vi "Autonomous Independent.vi"   [LabVIEW 2017]
doc: "This VI is called when autonomous begins, and will automatically be terminated when autonomous ends. You can carry out timed or sensor driven robot movement independently without needing to return to the caller."
uses:
  <vilib>/Rock Robotics/WPI/Solenoid/WPI_SolenoidValue.ctl
  <vilib>/Rock Robotics/WPI/SafetyOutput/WPI_SafetyOutputConfigMenu.ctl
  <vilib>/Rock Robotics/WPI/Utilities/WPI_GetSetVariantRefNum.vi
  <vilib>/Rock Robotics/WPI/Solenoid/WPI_SolenoidSetEnum.vi
  <vilib>/Rock Robotics/WPI/RobotDrive/WPI_RobotDriveArcadeDrive_Standard(NoSaturation).vi
  <vilib>/Rock Robotics/Network Tables/NT Read String.vi
  <vilib>/Rock Robotics/Network Tables/NT Write Numeric Array.vi
panel:
  # "Be sure to right-click and choose Data Operations>>Make Current Value default if you want to save the array values with the VI"
types:
  T1 = typedef "WPI_JoystickDevRef.ctl" = cluster{"Device":T2}
  T2 = typedef "WPI_JoystickDeviceEnum.ctl" = enum16{"USB 0", "USB 1", "USB 2", "USB 3", "USB 4", "USB 5"}
  T3 = typedef "WPI_SolenoidDevRef.ctl" = cluster{"DevStatus":errorcluster, "Pneumatics Control Module":u8, "Forward Solenoid Channel":T4, "Reverse Solenoid Channel":T4}
  T4 = typedef "WPI_SolenoidChannel.ctl" = enum8{"Solenoid 0", "Solenoid 1", "Solenoid 2", "Solenoid 3", "Solenoid 4", "Solenoid 5", "Solenoid 6", "Solenoid 7", "Invalid"}
  T5 = typedef "WPI_MotorControlDeviceRef.ctl" = cluster{"DeviceStatus":errorcluster, "Type":T6, "PWM":cluster{"PWM Channel":T7, "DeadBand":T8}, "CAN":cluster{"Device Number":u8, "SetOutput VI Ref":variant, "GetOutput VI Ref":variant, "Enable VI Ref":variant, "Disable VI Ref":variant, "Data":variant}, "Invert":bool, "DIO PWM":cluster{"PWM \"Enable\" Channel":T7, "DIOChannel":T9, "PWM Rate":dbl}}
  T6 = typedef "WPI_MotorControlType.ctl" = enum16{"PWM", "CAN", "DIO PWM"}
  T7 = typedef "FPGA_DIOPWMChannel.ctl" = enum8{"PWM 0", "PWM 1", "PWM 2", "PWM 3", "PWM 4", "PWM 5", "PWM 6", "PWM 7", "PWM 8", "PWM 9", "PWM MXP 0", "PWM MXP 1", "PWM MXP 2", "PWM MXP 3", "PWM MXP 4", "PWM MXP 5", "PWM MXP 6", "PWM MXP 7", "PWM MXP 8", "PWM MXP 9", "Invalid"}
  T8 = typedef "WPI_PWMDeadband.ctl" = cluster{"Name":string, "maxPositivePwm":i32, "minPositivePwm":i32, "centerPwm":i32, "maxNegativePwm":i32, "minNegativePwm":i32, "angularRange":u16}
  T9 = typedef "FPGA_DIOChannel.ctl" = enum8{"DIO 0", "DIO 1", "DIO 2", "DIO 3", "DIO 4", "DIO 5", "DIO 6", "DIO 7", "DIO 8", "DIO 9", "DIO MXP 0", "DIO MXP 1", "DIO MXP 2", "DIO MXP 3", "DIO MXP 4", "DIO MXP 5", "DIO MXP 6", "DIO MXP 7", "DIO MXP 8", "DIO MXP 9", "DIO MXP 10", "DIO MXP 11", "DIO MXP 12", "DIO MXP 13", "DIO MXP 14", "DIO MXP 15", "SPI Port CS1", "SPI Port CS2", "SPI Port CS3", "SPI Port MISO", "SPI Port MOSI", "Invalid"}
  T10 = typedef "WPI_RobotDriveDevRef.ctl" = cluster{"DevStatus":errorcluster, "Motors[]":T5[], "Square Inputs":bool, "Max Output":dbl}
  T11 = typedef "WPI_SolenoidValue.ctl" = enum16{"Off", "On", "Forward", "Reverse"}
  T12 = typedef "WPI_SafetyOutputConfigMenu.ctl" = enum16{"Enable", "Disable"}
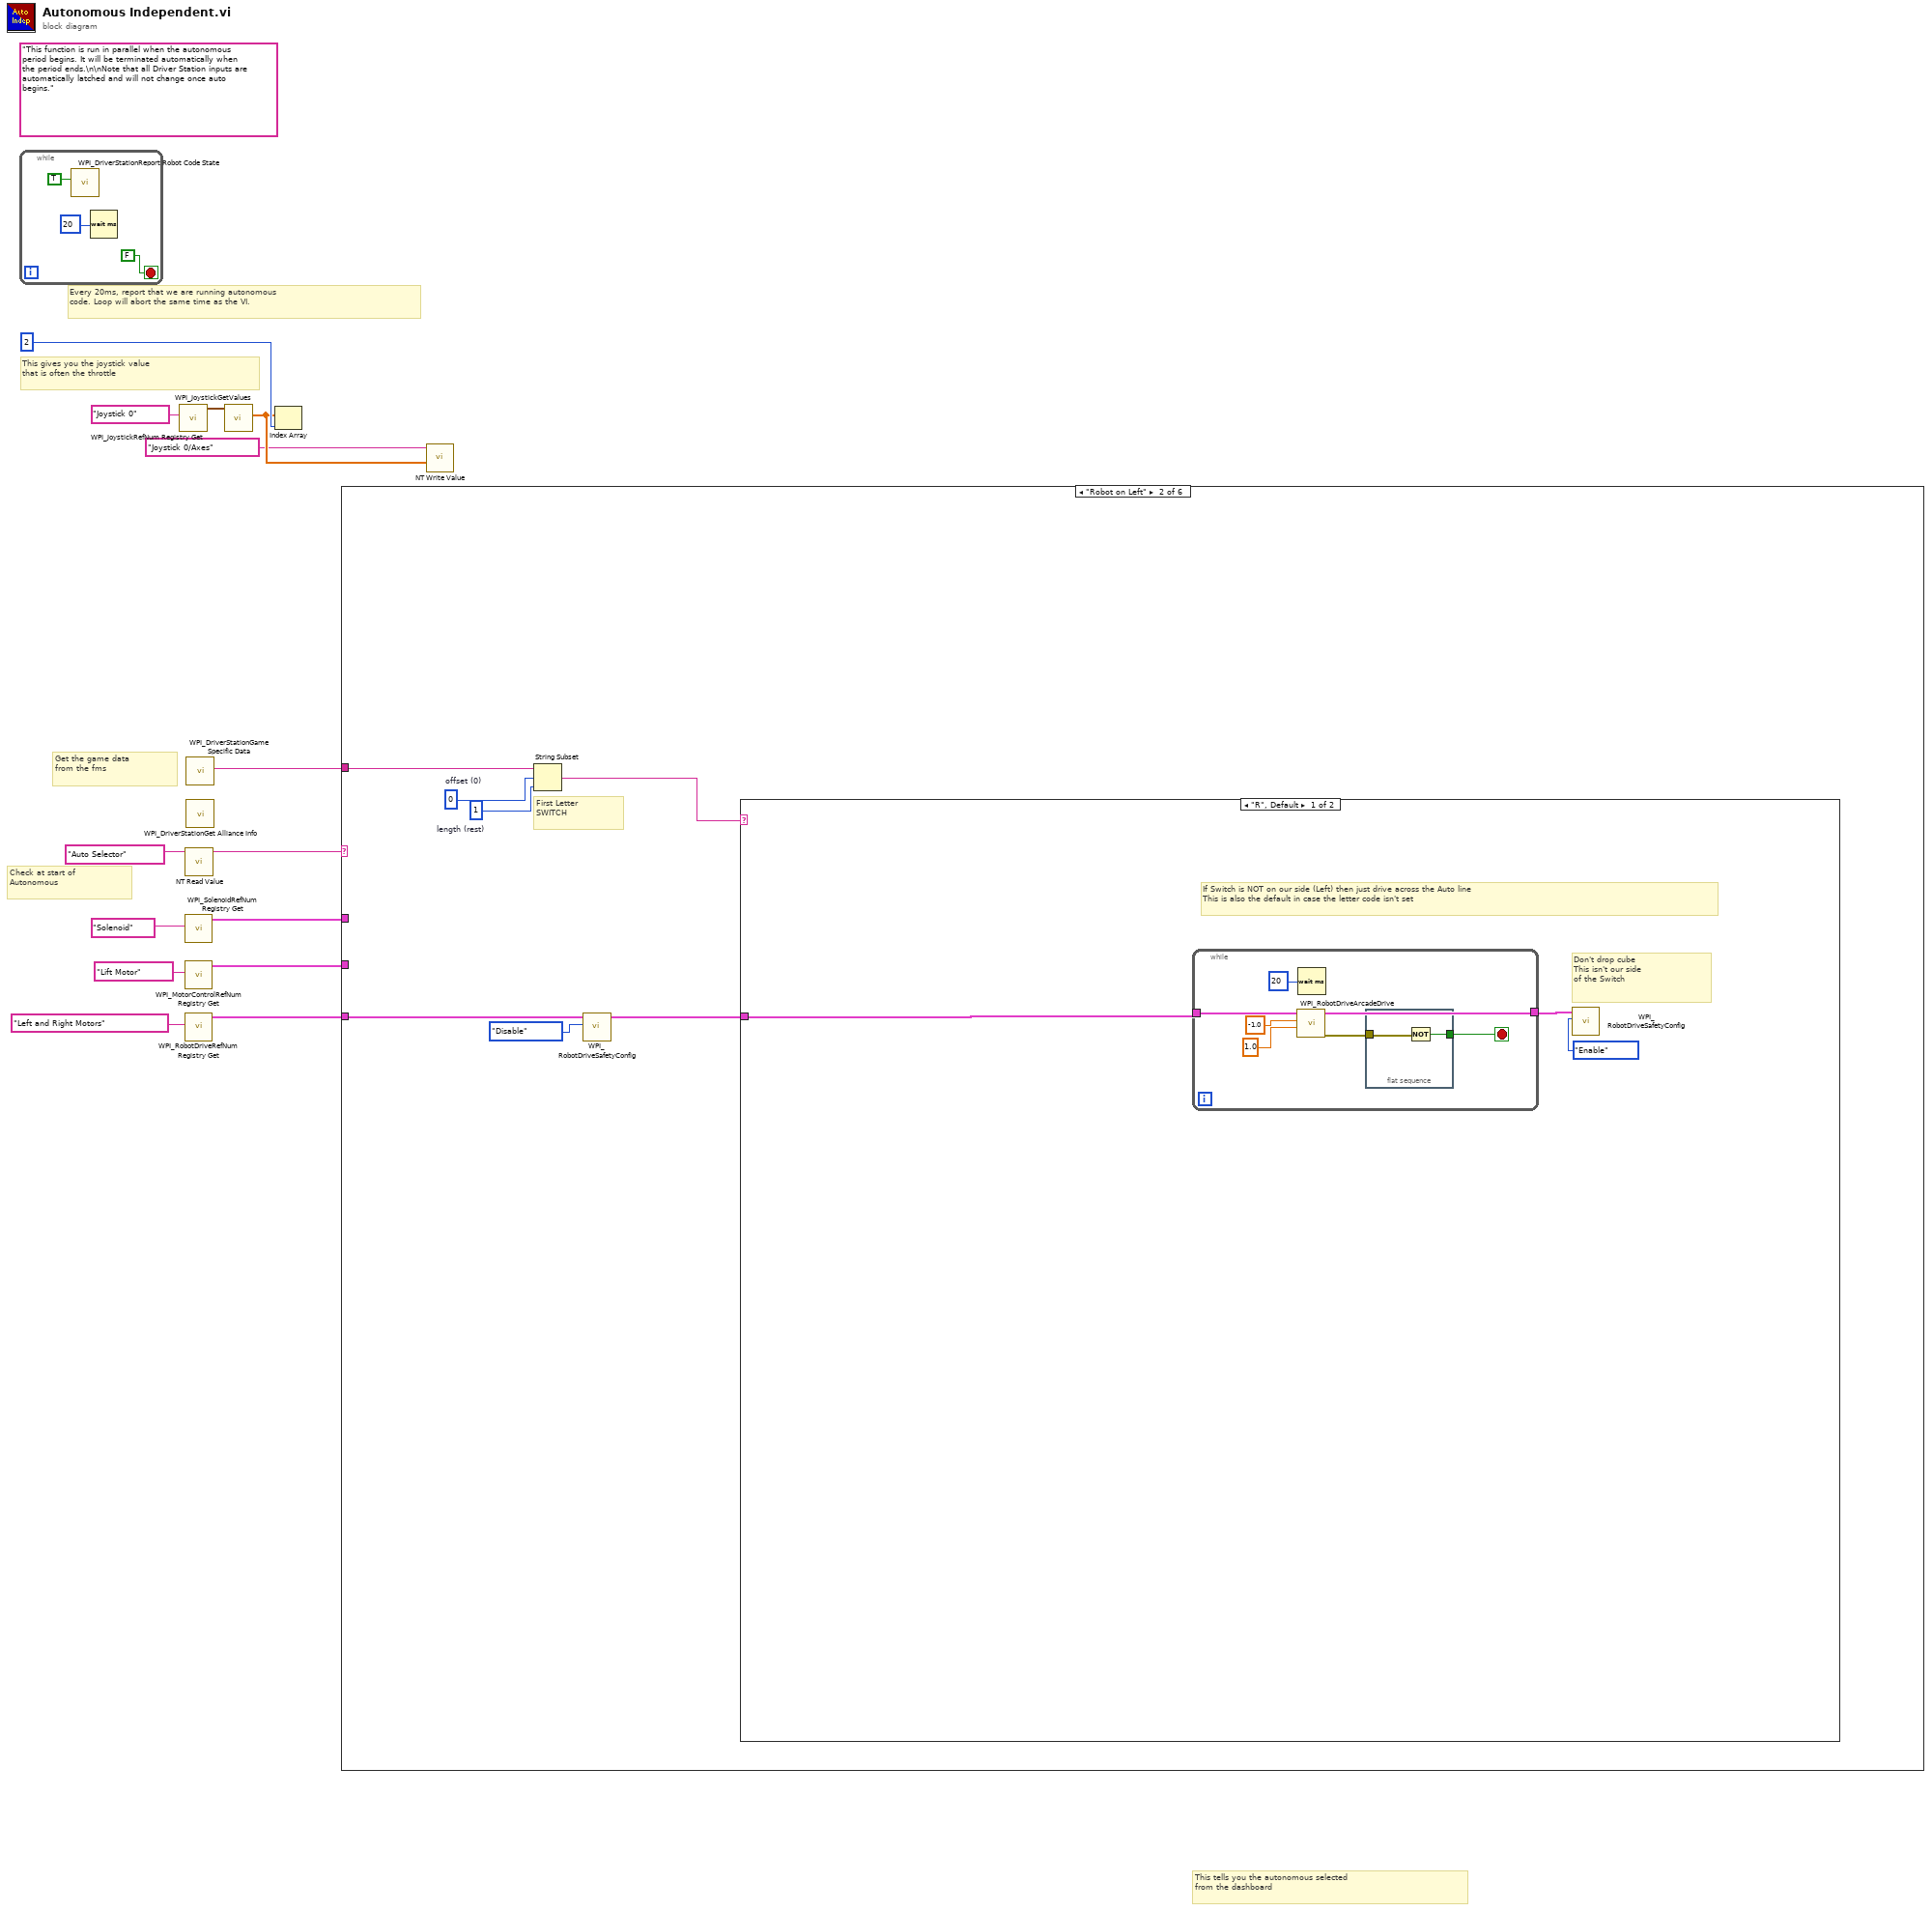
[diagram p0: block diagram]
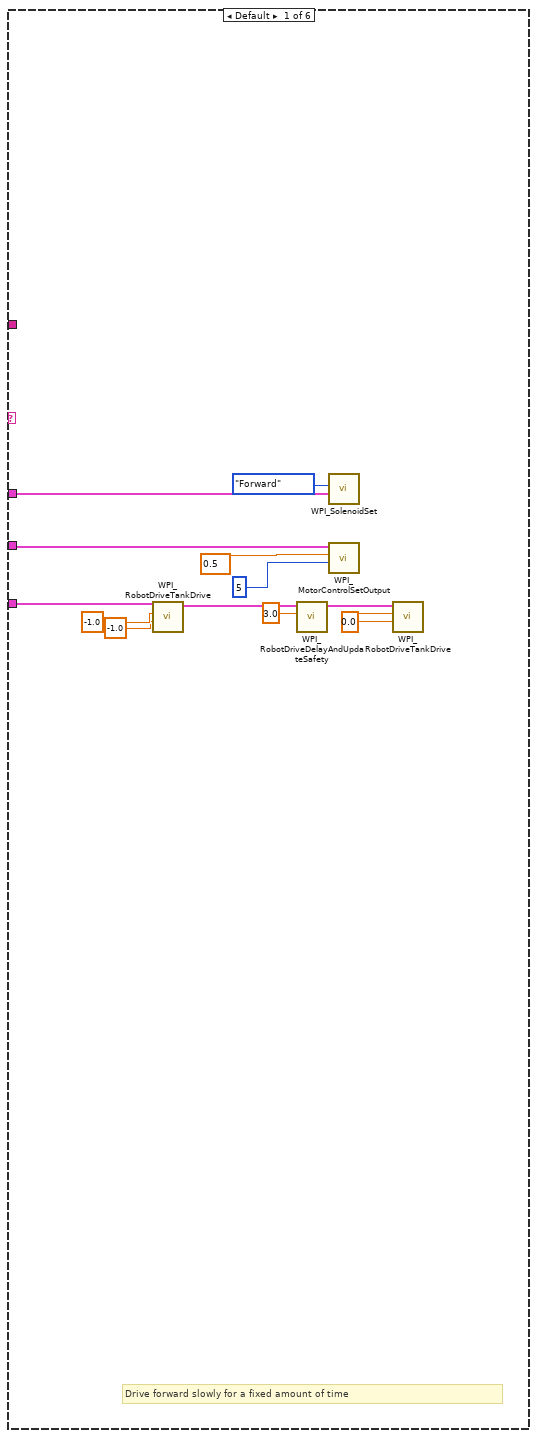
[diagram p2: hidden frame]
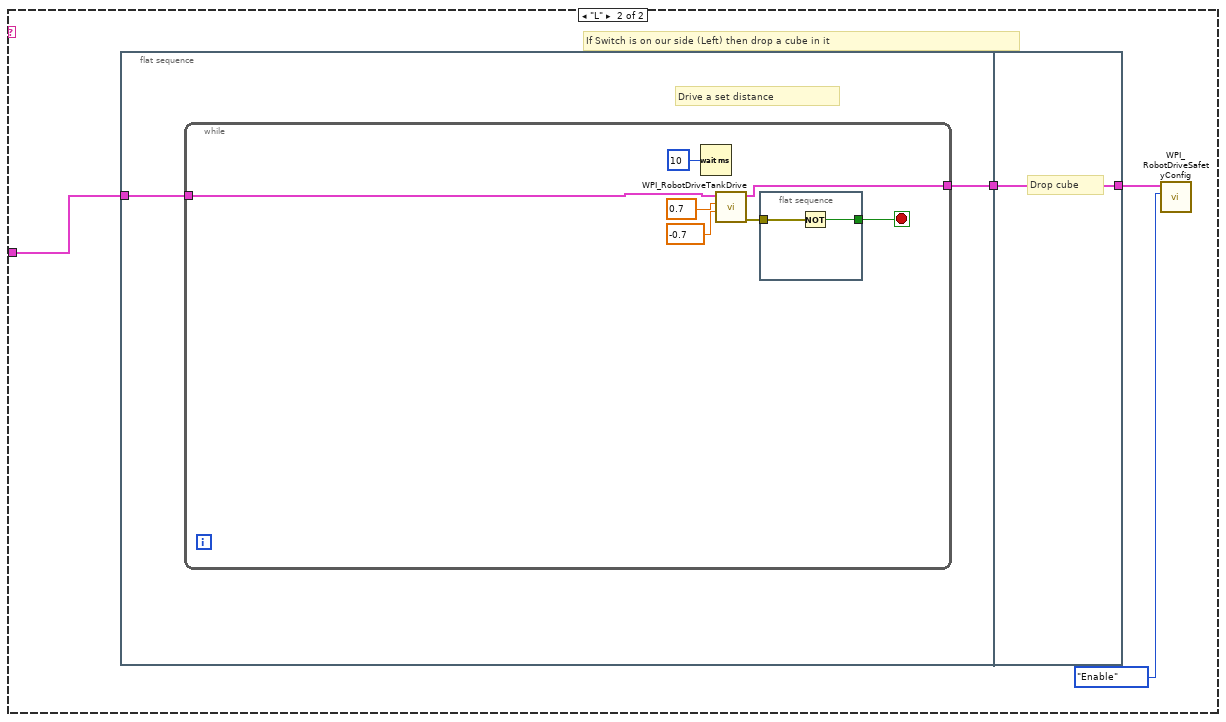
[diagram p3: hidden frame]
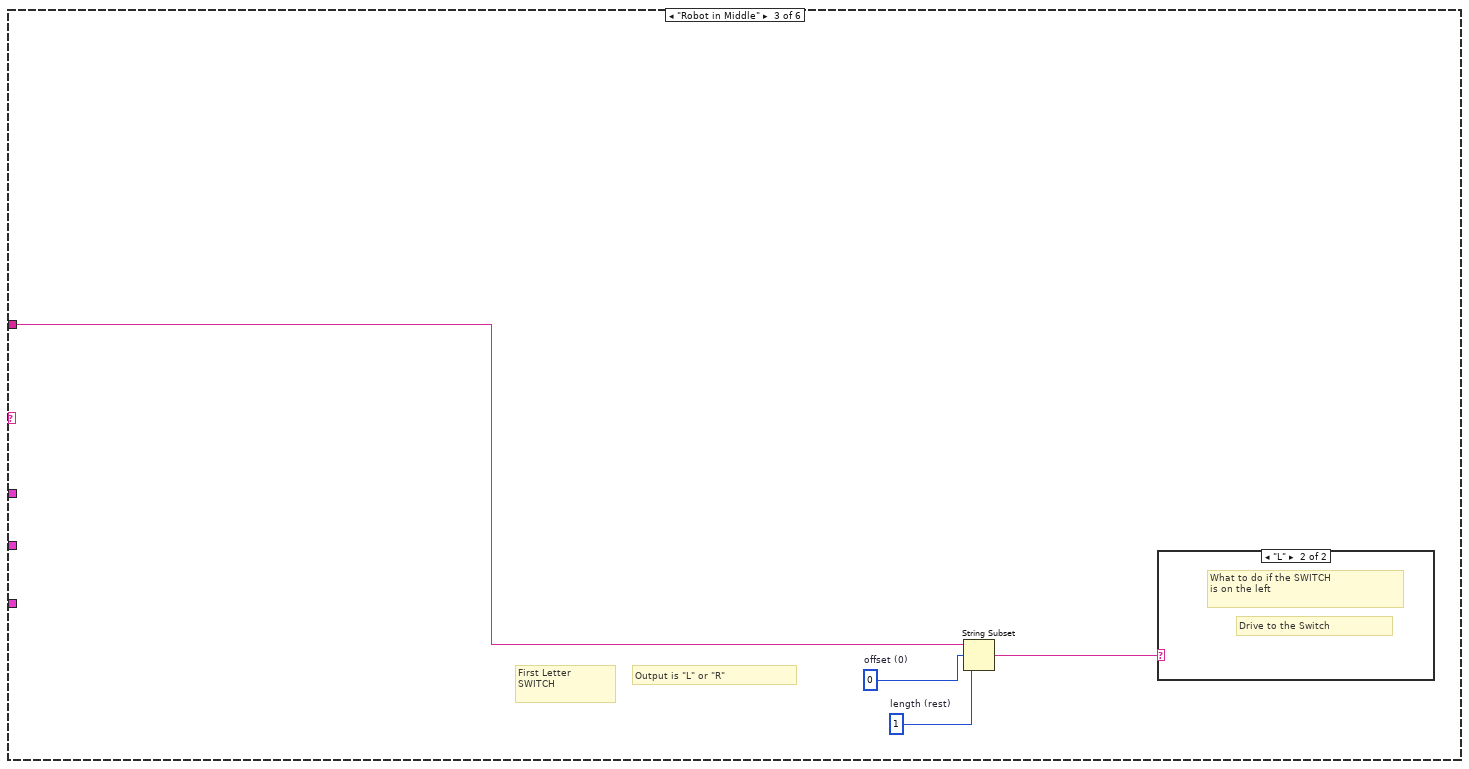
[diagram p4: hidden frame]
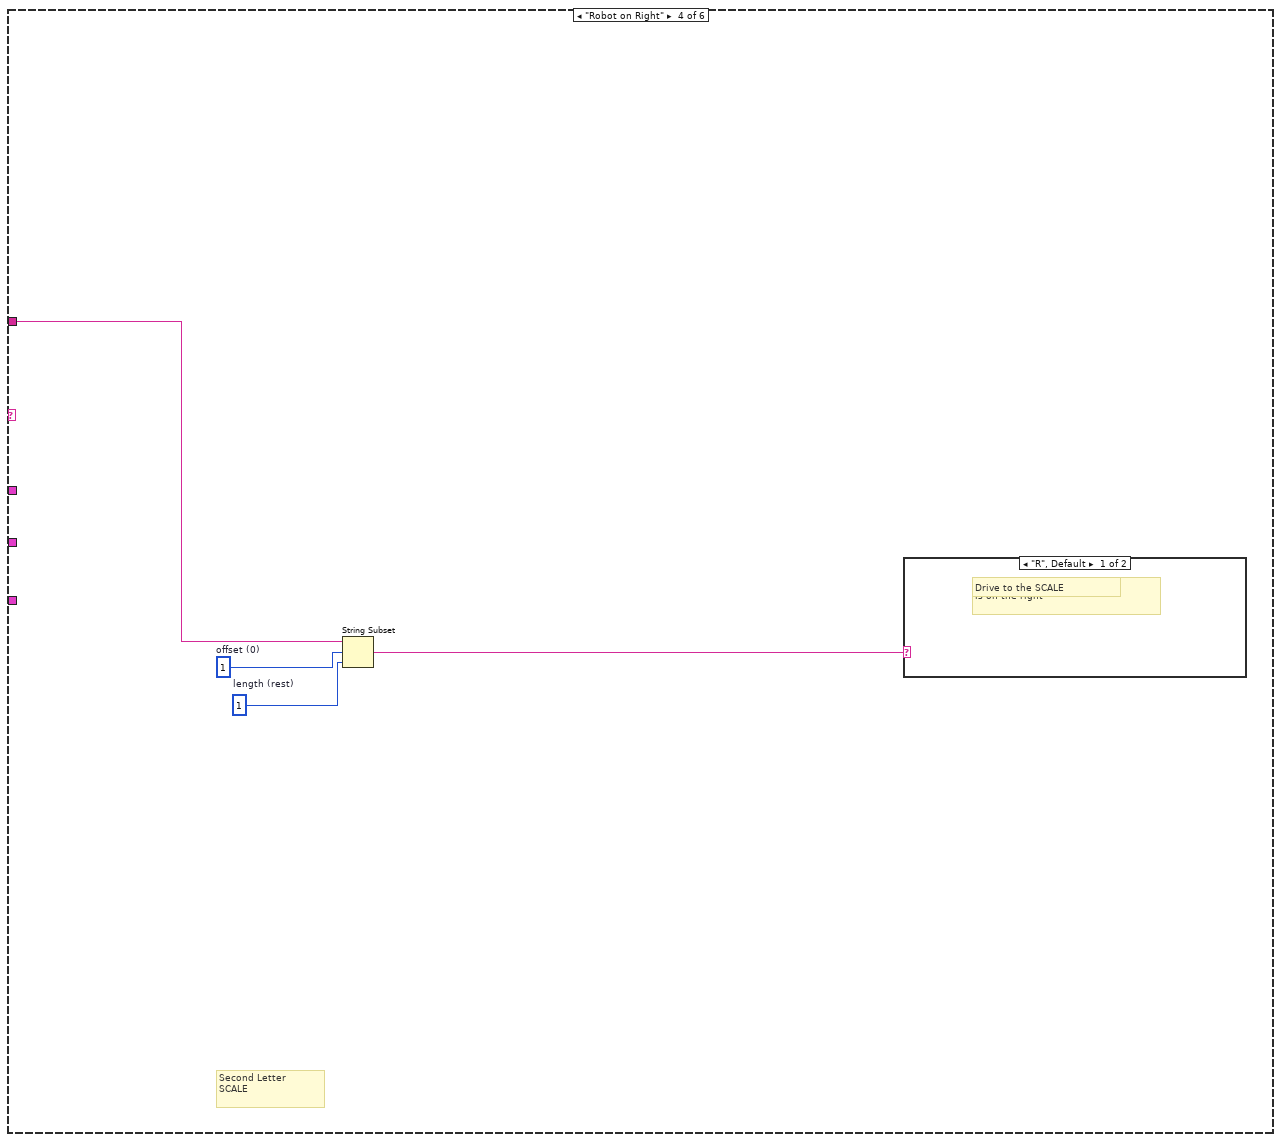
[diagram p6: hidden frame]
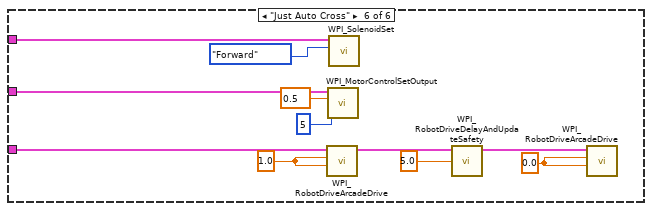
[diagram p9: hidden frame]
diagram:
  (unwired) "This function is run in parallel when the autonomous period begins. It will be terminated automatically when the period ends.\n\nNote that all Driver Station inputs are automatically latched and will not change once auto begins."
  # "Get the game data\nfrom the fms"
  # "This gives you the joystick value\nthat is often the throttle"
  # "Check at start of\nAutonomous"
  # "This tells you the autonomous selected\nfrom the dashboard"
  # "Every 20ms, report that we are running autonomous\ncode. Loop will abort the same time as the VI."
  n1 = while {
    stop <- FALSE stop-if-true
    n2 = call <vilib>:"WPI_DriverStationReport Robot Code State.vi"("Autonomous"=TRUE) -> ()  [unwired: 10 in, 1 out]
    n3 = Wait (ms)(milliseconds to wait=u32 20) -> ()  [unwired: 1 out]
  }
  n4 = call <vilib>:"WPI_JoystickRefNum Registry Get.vi"("refnum name"="Joystick 0") -> ("JoystickDevRef"=w8:T1)  [unwired: 1 in, 9 out]
  n5 = call <vilib>:"WPI_SolenoidRefNum Registry Get.vi"("refnum name"="Solenoid") -> ("SolenoidDevRef"=w3:T3)  [unwired: 9 in, 1 out]
  n6 = call <vilib>:"WPI_MotorControlRefNum Registry Get.vi"("refnum name"="Lift Motor") -> ("MotorControlDevRef"=w1:T5)  [unwired: 9 in, 1 out]
  n7 = call <vilib>:"WPI_RobotDriveRefNum Registry Get.vi"("refnum name"="Left and Right Motors") -> ("RobotDriveDevRef"=w11:T10)  [unwired: 1 in, 9 out]
  n8 = call-poly <vilib>:"NT Read Value.vi"("Name"="Auto Selector") -> ("String"=w13:string)  [unwired: 9 in, 1 out]
  n9 = call <vilib>:"WPI_DriverStationGame Specific Data.vi"() -> ("Game Specific Data"=w10:string)  [unwired: 11 in]
  n10 = call <vilib>:"WPI_DriverStationGet Alliance Info.vi"() -> ()  [unwired: 12 out]
  n11 = call <vilib>:"WPI_JoystickGetValues.vi"("JoystickDevRef"=w8) -> ("Axes"=w6:dbl[])  [unwired: 6 in, 4 out]
  n12 = Index Array(array=w6, index=2) -> ()  [unwired: 1 out]
  n13 = case shown="\"Robot on Left\"" w13 {
    tunnel: w11 -> [w23 w33 _ _ _ w79]
    tunnel: w10 -> [_ w30 w65 w69 _ _]
    tunnel: w3 -> [w19 _ _ _ _ w78]
    tunnel: w1 -> [w18 _ _ _ _ w76]
    frame Default {
      w24 = 0.0 ("X axis value")
      # "Drive forward slowly for a fixed amount of time"
      n14 = call <vilib>:"WPI_RobotDriveTankDrive.vi"("Right axis value"=-1.0 ("Y axis value"), "Left axis value"=-1.0 ("X axis value"), "RobotDriveDevRef"=w23) -> ("RobotDriveDevRef"=w29:T10)  [unwired: 6 in, 2 out]
      n15 = call <vilib>:"WPI_RobotDriveDelayAndUpdateSafety.vi"("Delay (s)"=3.0, "RobotDriveDevRef"=w29) -> ("RobotDriveDevRef 2"=w25:T10)  [unwired: 8 in, 1 out]
      n16 = call-poly <vilib>:"WPI_SolenoidSet.vi"("Value"=WPI_SolenoidValue."Forward", "SolenoidDevRef"=w19) -> ()  [unwired: 8 in, 2 out]
      n17 = call <vilib>:"WPI_MotorControlSetOutput.vi"("options"=u8 5, "Output"=0.5, "MotorControlDevRef"=w18) -> ()  [unwired: 6 in, 3 out]
      n18 = call <vilib>:"WPI_RobotDriveTankDrive.vi"("Right axis value"=w24, "Left axis value"=w24, "RobotDriveDevRef"=w25) -> ()  [unwired: 6 in, 3 out]
    }
    frame "Robot on Left" {
      w36 = 1  # length (rest)
      w35 = 0  # offset (0)
      # "First Letter\nSWITCH"
      n19 = String Subset(string=w30, offset (0)=w35, length (rest)=w36) -> (substring=w34:string)
      n20 = call <vilib>:"WPI_RobotDriveSafetyConfig.vi"("mode"=WPI_SafetyOutputConfigMenu."Disable", "RobotDriveDevRef"=w33) -> ("RobotDriveDevRef"=w32:T10)  [unwired: 8 in, 1 out]
      n21 = case shown="\"R\", Default" w34 {
        tunnel: w32 -> [w39 w51]
        frame "R", Default {
          # "Don't drop cube\nThis isn't our side\nof the Switch"
          # "If Switch is NOT on our side (Left) then just drive across the Auto line\nThis is also the default in case the letter code isn't set"
          n22 = while {
            tunnel: w39 -> [w43]
            tunnel: [w42] -> w37
            stop <- w46 stop-if-true
            n23 = call-poly <vilib>:"WPI_RobotDriveArcadeDrive.vi"("Y axis value"=1.0, "X axis value"=-1.0, "RobotDriveDevRef"=w43) -> ("error out"=w41:errorcluster, "RobotDriveDevRef"=w42:T10)  [unwired: 6 in, 1 out]
            n24 = Wait (ms)(milliseconds to wait=u32 20) -> ()  [unwired: 1 out]
            n25 = flat-sequence {
              tunnel: [w48] -> w46
              tunnel: w41 -> [w47]
              frame #0 {
                n26 = Not(x=w47) -> (.not. x?=w48:bool)
              }
            }
          }
          n27 = call <vilib>:"WPI_RobotDriveSafetyConfig.vi"("mode"=WPI_SafetyOutputConfigMenu."Enable", "RobotDriveDevRef"=w37) -> ()  [unwired: 8 in, 2 out]
        }
        frame "L" {
          # "If Switch is on our side (Left) then drop a cube in it"
          n28 = flat-sequence {
            tunnel: [w54] -> w52
            tunnel: w51 -> [w53]
            tunnel: w52 -> [w64]
            tunnel: [w64] -> w49
            frame #0 {
              # "Drive a set distance"
              n29 = while {
                tunnel: w53 -> [w58]
                tunnel: [w57] -> w54
                stop <- w61 stop-if-true
                n30 = Wait (ms)(milliseconds to wait=u32 10) -> ()  [unwired: 1 out]
                n31 = call <vilib>:"WPI_RobotDriveTankDrive.vi"("Right axis value"=-0.7, "Left axis value"=0.7 ("X axis value"), "RobotDriveDevRef"=w58) -> ("error out"=w56:errorcluster, "RobotDriveDevRef"=w57:T10)  [unwired: 6 in, 1 out]
                n32 = flat-sequence {
                  tunnel: [w63] -> w61
                  tunnel: w56 -> [w62]
                  frame #0 {
                    n33 = Not(x=w62) -> (.not. x?=w63:bool)
                  }
                }
              }
            }
            frame #1 {
              # "Drop cube"
            }
          }
          n34 = call <vilib>:"WPI_RobotDriveSafetyConfig.vi"("mode"=WPI_SafetyOutputConfigMenu."Enable", "RobotDriveDevRef"=w49) -> ()  [unwired: 8 in, 2 out]
        }
      }
    }
    frame "Robot in Middle" {
      w68 = 1  # length (rest)
      w67 = 0  # offset (0)
      # "Output is \"L\" or \"R\""
      # "First Letter\nSWITCH"
      n35 = String Subset(string=w65, offset (0)=w67, length (rest)=w68) -> (substring=w66:string)
      n36 = case shown="\"L\"" w66 {
        frame "R", Default {
          # "What to do if the SWITCH\nis on the right"
          # "Drive to the SWITCH"
        }
        frame "L" {
          # "Drive to the Switch"
          # "What to do if the SWITCH\nis on the left"
        }
      }
    }
    frame "Robot on Right" {
      w71 = 1  # length (rest)
      w70 = 1  # offset (0)
      # "Second Letter\nSCALE"
      n37 = String Subset(string=w69, offset (0)=w70, length (rest)=w71) -> (substring=w72:string)
      n38 = case shown="\"R\", Default" w72 {
        frame "R", Default {
          # "What to do if the SCALE\nis on the right"
          # "Drive to the SCALE"
        }
        frame "L" {
          # "What to do if the SCALE\nis on the left"
          # "Drive to the SCALE"
        }
      }
    }
    frame "Do Nothing" {
      # "In case something is broken"
    }
    frame "Just Auto Cross" {
      w80 = 0.0 ("X axis value")
      w73 = 1.0 ("X axis value")
      n39 = call-poly <vilib>:"WPI_RobotDriveArcadeDrive.vi"("Y axis value"=w73, "X axis value"=w73, "RobotDriveDevRef"=w79) -> ("RobotDriveDevRef"=w82:T10)  [unwired: 6 in, 2 out]
      n40 = call <vilib>:"WPI_MotorControlSetOutput.vi"("options"=u8 5, "Output"=0.5, "MotorControlDevRef"=w76) -> ()  [unwired: 6 in, 3 out]
      n41 = call-poly <vilib>:"WPI_SolenoidSet.vi"("Value"=WPI_SolenoidValue."Forward", "SolenoidDevRef"=w78) -> ()  [unwired: 8 in, 2 out]
      n42 = call <vilib>:"WPI_RobotDriveDelayAndUpdateSafety.vi"("Delay (s)"=5.0, "RobotDriveDevRef"=w82) -> ("RobotDriveDevRef 2"=w83:T10)  [unwired: 8 in, 1 out]
      n43 = call-poly <vilib>:"WPI_RobotDriveArcadeDrive.vi"("Y axis value"=w80, "X axis value"=w80, "RobotDriveDevRef"=w83) -> ()  [unwired: 6 in, 3 out]
    }
  }
  n44 = call-poly <vilib>:"NT Write Value.vi"("Numeric Array"=w6, "Name"="Joystick 0/Axes") -> ()  [unwired: 9 in, 1 out]
